vi "DIAcqSubVI.vi"(8 "error in (no error)":errorcluster, 11 "Data Cluster In":T1) -> (0 "error out":errorcluster, 2 "data":bool[](array[boolean]), 3 "Data Cluster Out":T1)   [LabVIEW 2017]
doc: "Acquires data from digital inputs of DAQ."
uses:
  Controls/ShiftRegisterCluster.ctl
  <vilib>/DAQmx/read.llb/DAQmx Read (Digital 1D Bool NChan 1Samp 1Line).vi
  <vilib>/DAQmx/miscellaneous.llb/DAQmx Fill In Error Info.vi
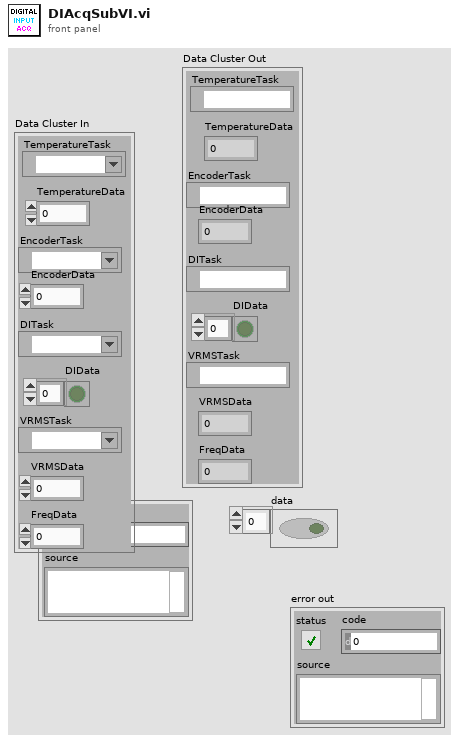
[diagram p1: front panel]
types:
  T1 = typedef "ShiftRegisterCluster.ctl" = cluster{"TemperatureTask":refnum<k21>, "TemperatureData":dbl, "EncoderTask":refnum<k21>, "EncoderData":dbl, "DITask":refnum<k21>, "DIData":bool[], "VRMSTask":refnum<k21>, "VRMSData":dbl, "FreqData":dbl}
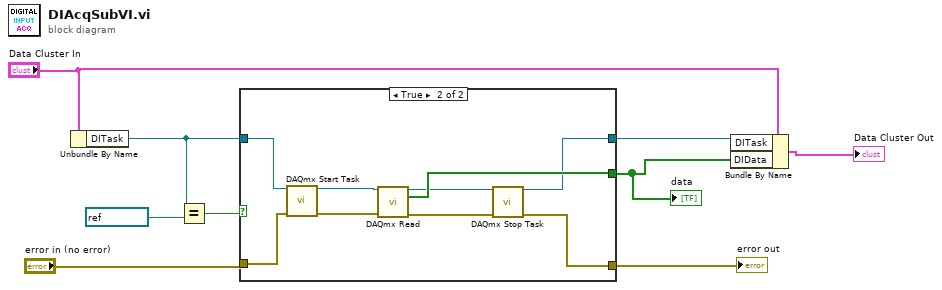
[diagram p0: block diagram]
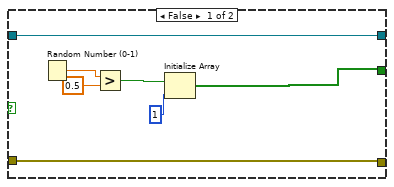
[diagram p2: hidden frame]
diagram:
  n1 = Unbundle By Name("Data Cluster In") -> ("DITask"=w6:refnum<k21>)
  n2 = Equal?(x=w6, y=refnum<k21> "DITask" ("DAQmx Task Name")) -> (x = y?=w4:bool)
  n3 = case shown="True" w4 {
    tunnel: w6 -> [w16 w25]
    tunnel: [w11 w24] -> w3
    tunnel: [w12 w22] -> w9
    tunnel: "error in (no error)" -> [w12 w18]
    tunnel: [w16 w17] -> w7
    frame False {
      n4 = Random Number (0-1)() -> (number: 0 to 1=w15:dbl)
      n5 = Greater?(x=w15, y=0.5) -> (0:w13:bool)
      n6 = Initialize Array(w13, 1 ("dimension size")) -> (w11:bool[])
    }
    frame True {
      n7 = call <vilib>:"DAQmx Start Task.vi"("task/channels in"=w25, "error in"=w18) -> ("task out"=w23:refnum<k21>, "error out"=w19:errorcluster)  [unwired: 12 in]
      n8 = call-poly <vilib>:"DAQmx Read.vi"("task/channels in"=w23, "error in"=w19) -> ("task out"=w20:refnum<k21>, "data"=w24:bool[], "error out"=w21:errorcluster)  [unwired: 11 in]
      n9 = call <vilib>:"DAQmx Stop Task.vi"("task/channels in"=w20, "error in"=w21) -> ("task out"=w17:refnum<k21>, "error out"=w22:errorcluster)  [unwired: 12 in]
    }
  }
  "error out" <- w9
  "data" <- w3
  n10 = Bundle By Name(cluster="Data Cluster In", "DITask"=w7, "DIData"=w3) -> (→"Data Cluster Out":T1)
